vi "DSF.Execution.Plugin.Get ID.vi"(8 "error in (no error)":errorcluster, 11 "Plugin in":refnum<class "DSF.Execution.Plugin.lvclass">) -> (0 "error out":errorcluster, 2 "id":i32, 3 "Plugin out":refnum<class "DSF.Execution.Plugin.lvclass">)   [LabVIEW 2016, in "DSF.Execution.lvlib" / "DSF.Execution.Plugin.lvclass"]
uses:
  DSF.Execution.Plugin.lvclass
  DSF.Execution.Plugin.lvclass/DSF.Execution.Plugin.ctl
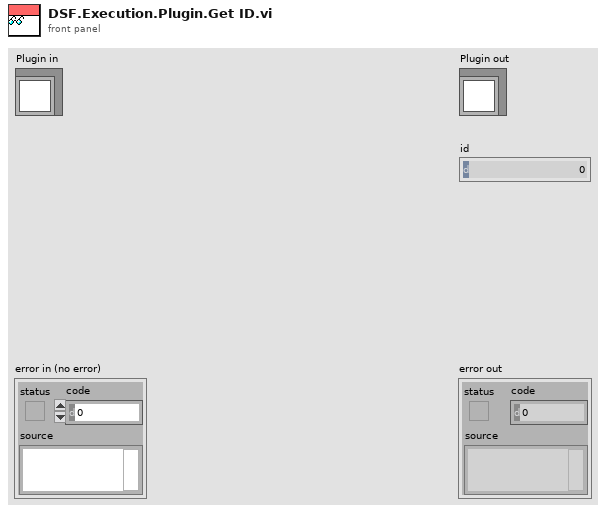
[diagram p1: front panel]
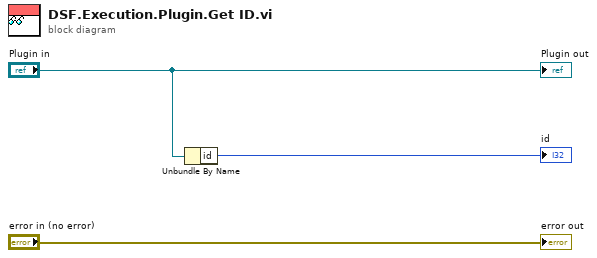
[diagram p0: block diagram]
diagram:
  n1 = Unbundle By Name("Plugin in") -> ("id"=→"id":i32)
  "error out" <- "error in (no error)"
  "Plugin out" <- "Plugin in"
